vi "Stop Core.vi"(10 "final error code":i32, 11 "Mediator in":refnum<class "Mediator.lvclass">) -> (3 "Mediator out":refnum<class "Mediator.lvclass">)   [LabVIEW 2015, in "Mediator.lvlib" / "Mediator.lvclass"]
doc: "(<B>Filename</B>: Actor Framework.lvlib:Actor.lvclass:Stop Core.vi)\n\nDefines what the actor does before it stops. Use the <B>final error code</B> input to determine whether the actor shut down in response to an error.\n\nBy default, this method does nothing. A descendant class may override it to define behavior, such as shutting down any processes the actor initiated in its override of the Actor Core method."
uses:
  Mediator.lvclass
  Mediator.lvclass/Mediator.ctl
  IMediator/IMediator/IMediator.lvclass
  TopicLookupTable/TopicLookupTable.lvclass
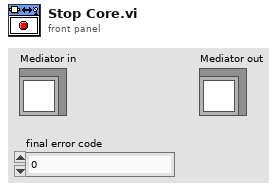
[diagram p1: front panel]
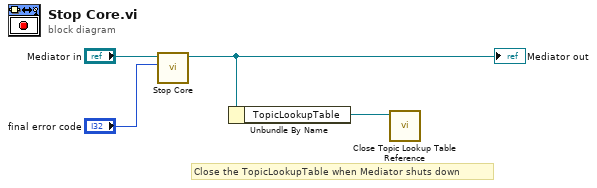
[diagram p0: block diagram]
diagram:
  # "Close the TopicLookupTable when Mediator shuts down"
  n1 = call-parent "Stop Core.vi"("final error code"="final error code", "Actor in"="Mediator in") -> ("Actor out"=w2:refnum<class "Mediator.lvclass">)  [unwired: 9 in]
  "Mediator out" <- w2
  n2 = Unbundle By Name(w2) -> ("TopicLookupTable"=w1:refnum<data-value>)
  n3 = call "Close Topic Lookup Table Reference.vi"("TopicLookupTable"=w1) -> ()  [unwired: 10 in, 1 out]
